vi "core_detect_boolean_edges.vi"(9 "tf input":bool) -> (0 "falling edge":bool, 2 "rising edge":bool)   [LabVIEW 2015]
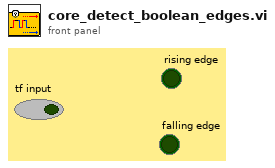
[diagram p1: front panel]
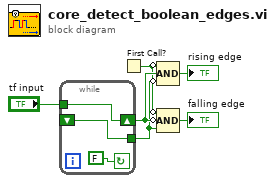
[diagram p0: block diagram]
diagram:
  n1 = while {
    tunnel: [w8] -> w5
    tunnel: "tf input" -> [w9]
    shift-left: _ -> [w8]
    shift-right: [w9] -> w6
    stop <- FALSE continue-if-true
  }
  n2 = First Call?() -> (First Call?: T/F=w1:bool)
  n3 = Compound Arithmetic op=AND(invert w1, w6, invert w5) -> (→"rising edge":bool)
  n4 = Compound Arithmetic op=AND(invert w1, invert w6, w5) -> (→"falling edge":bool)
